vi "Set dt on Variant.vi"(8 "error in (no error)":errorcluster, 10 "dt":dbl, 11 "Variant in":variant) -> (0 "error out":errorcluster, 1 "replaced":bool, 3 "Variant out":variant)   [LabVIEW 2020, in "Internal Comm Classes.lvlib" / "WPL Comm.lvclass"]
uses:
  WPL Comm.lvclass
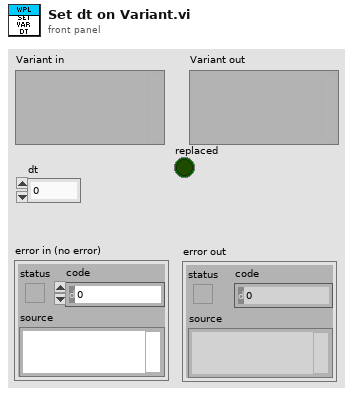
[diagram p1: front panel]
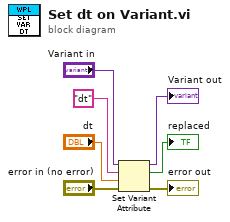
[diagram p0: block diagram]
diagram:
  n1 = Set Variant Attribute(Variant="Variant in", name="dt", value="dt", error in="error in (no error)") -> (Variant out=→"Variant out":variant, replaced=→"replaced":bool, error out=→"error out":errorcluster)
